vi "Find Mandingo.vi"(8 "Error In":errorcluster, 11 "Player Names":string[](array[string])) -> (0 "Error Out":errorcluster, 2 "Found Mandingo":bool, 3 "id Mandingo":dbl)   [LabVIEW 2015]
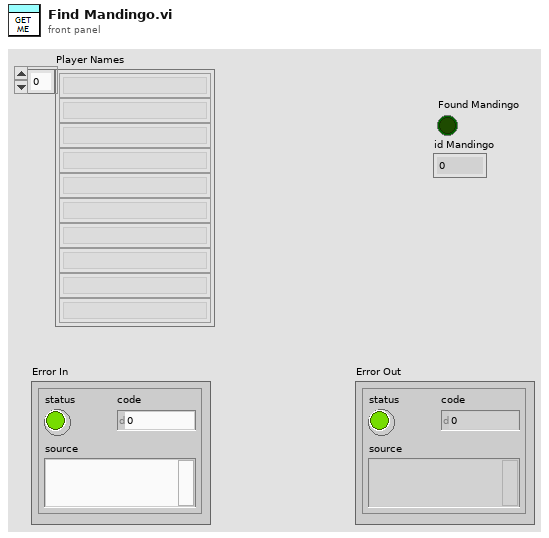
[diagram p1: front panel]
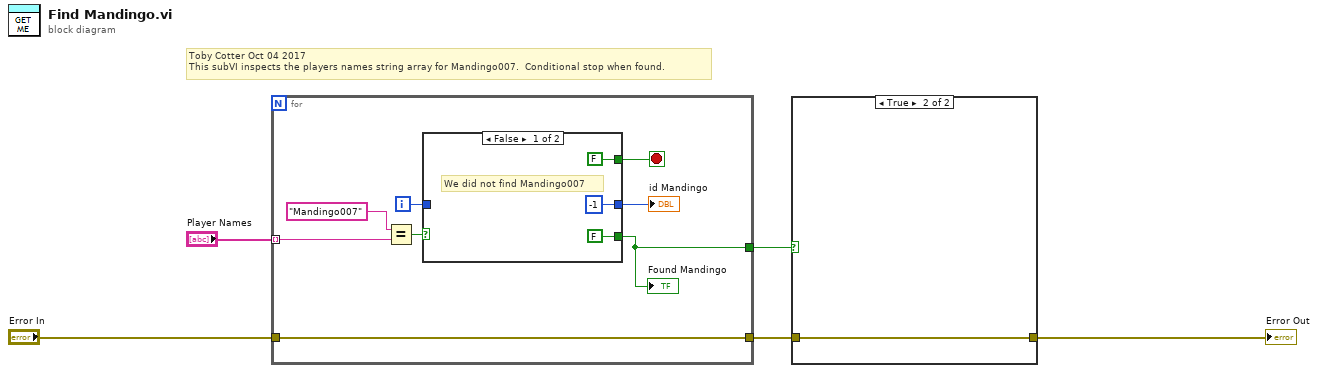
[diagram p0: block diagram]
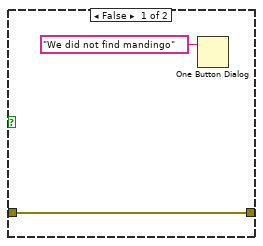
[diagram p2: hidden frame]
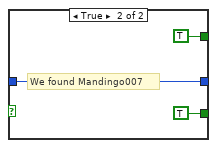
[diagram p3: hidden frame]
diagram:
  # "Toby Cotter Oct 04 2017\nThis subVI inspects the players names string array for Mandingo007.  Conditional stop when found."
  n1 = for {
    tunnel: "Player Names" -> [w13] mode=indexing
    tunnel: "Error In" -> [w7]
    tunnel: [w7] -> w3
    tunnel: [w6] -> w1
    i -> [w10]
    stop <- w8 stop-if-true
    n2 = Equal?(x="Mandingo007", y=w13) -> (x = y?=w11:bool)
    n3 = case shown="False" w11 {
      tunnel: [FALSE ("Found Mandingo") TRUE ("Found Mandingo")] -> w6
      tunnel: w10 -> [_ w18]
      tunnel: [-1 w18] -> w9
      tunnel: [FALSE ("Found Mandingo") TRUE ("Found Mandingo")] -> w8
      frame False {
        # "We did not find Mandingo007"
      }
      frame True {
        # "We found Mandingo007"
      }
    }
    "Found Mandingo" <- w6
    "id Mandingo" <- w9
  }
  n4 = case shown="True" w1 {
    tunnel: [w21 w22] -> w2
    tunnel: w3 -> [w21 w22]
    frame False {
      n5 = One Button Dialog(message="We did not find mandingo") -> ()  [unwired: 1 in, 1 out]
    }
    frame True {
    }
  }
  "Error Out" <- w2
